vi "PPMS_CREA_SECUENCIA_OLD.vi"(8 "error in (no error)":errorcluster) -> (0 "error out":errorcluster, 1 "Total":string[](array[string]), 2 "Pasos":i32, 3 "Secuencia":string[](array[string]))   [LabVIEW 2017]
uses:
  <vilib>/Utility/file.llb/Read From Spreadsheet File (string).vi
panel:
  out "subArray2D":string[][](array[string])
  out "Seq scans":string[](array[string])
  out "Seq final":string[](array[string])
  out "Seq inicial":string[](array[string])
  out "idxScanTi":i16
  out "idxScanFi":i16
  out "idxScanFf":i16
  out "idxScanTf":i16
  out "Array2D":string[][](array[string])
  out "Scan T":bool
  out "Scan F":bool
  in  "Salir":bool
  in  "Borra linea":bool
  in  "Grabar":bool
  in  "Cargar":bool
  out "SequenceFile":path
  in  "Command line (double click)":i32(listbox) caption="Válvulas"
  in  "Secuencia":i32(listbox)=-1
  # "Septiembre 2019 V1.2  a-sslcdms"
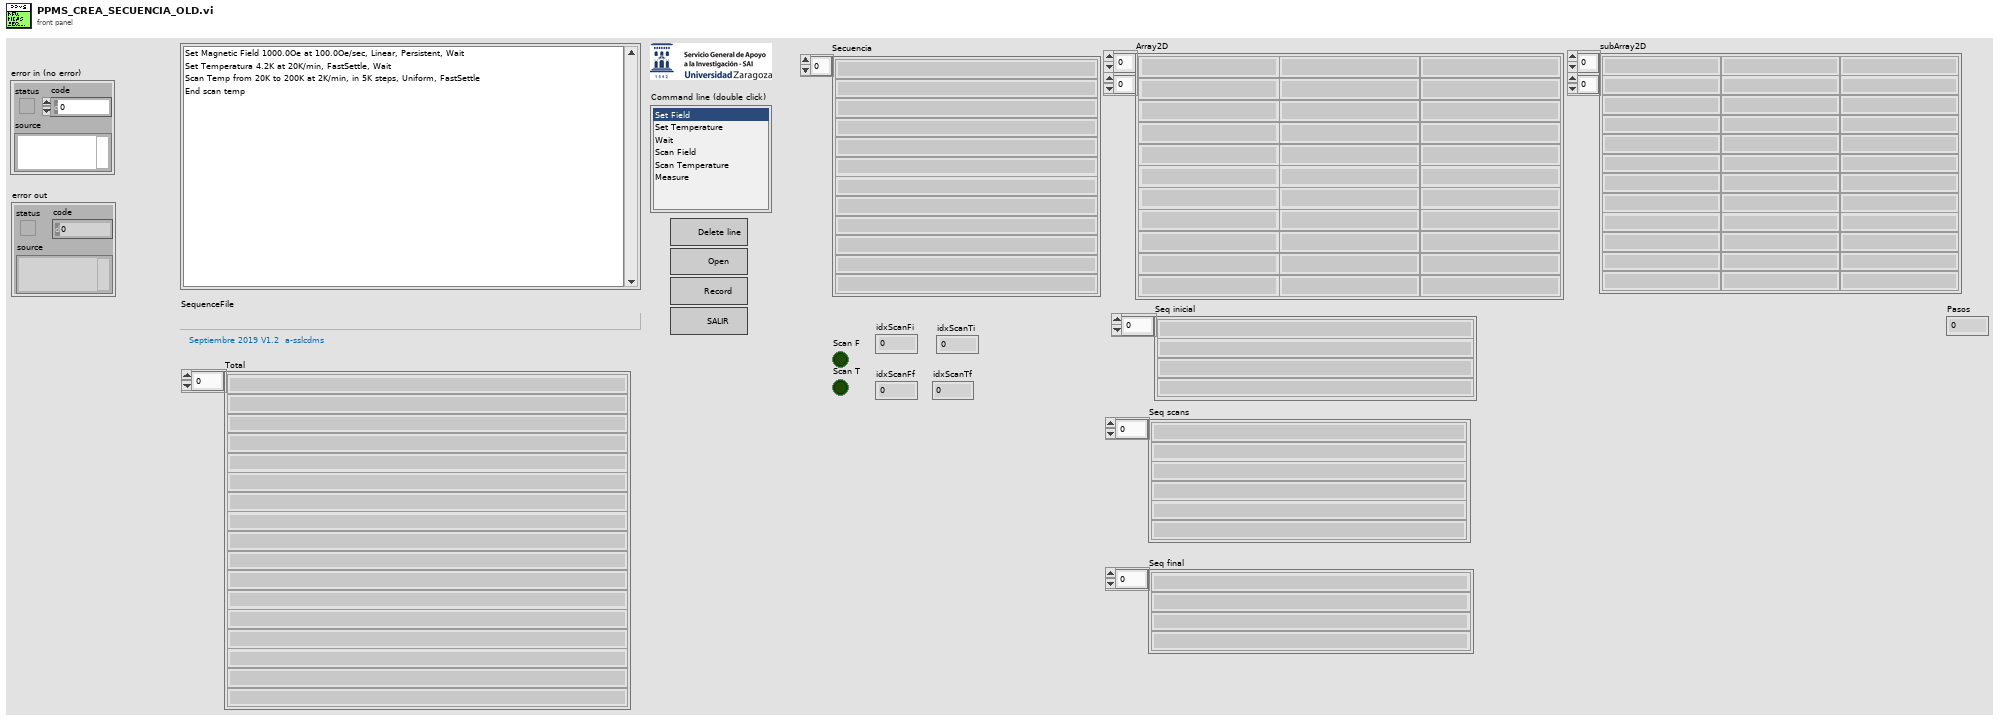
[diagram p1: front panel]
types:
  T1 = enum16{"open", "open or create", "create or replace", "create", "open (read only)"}
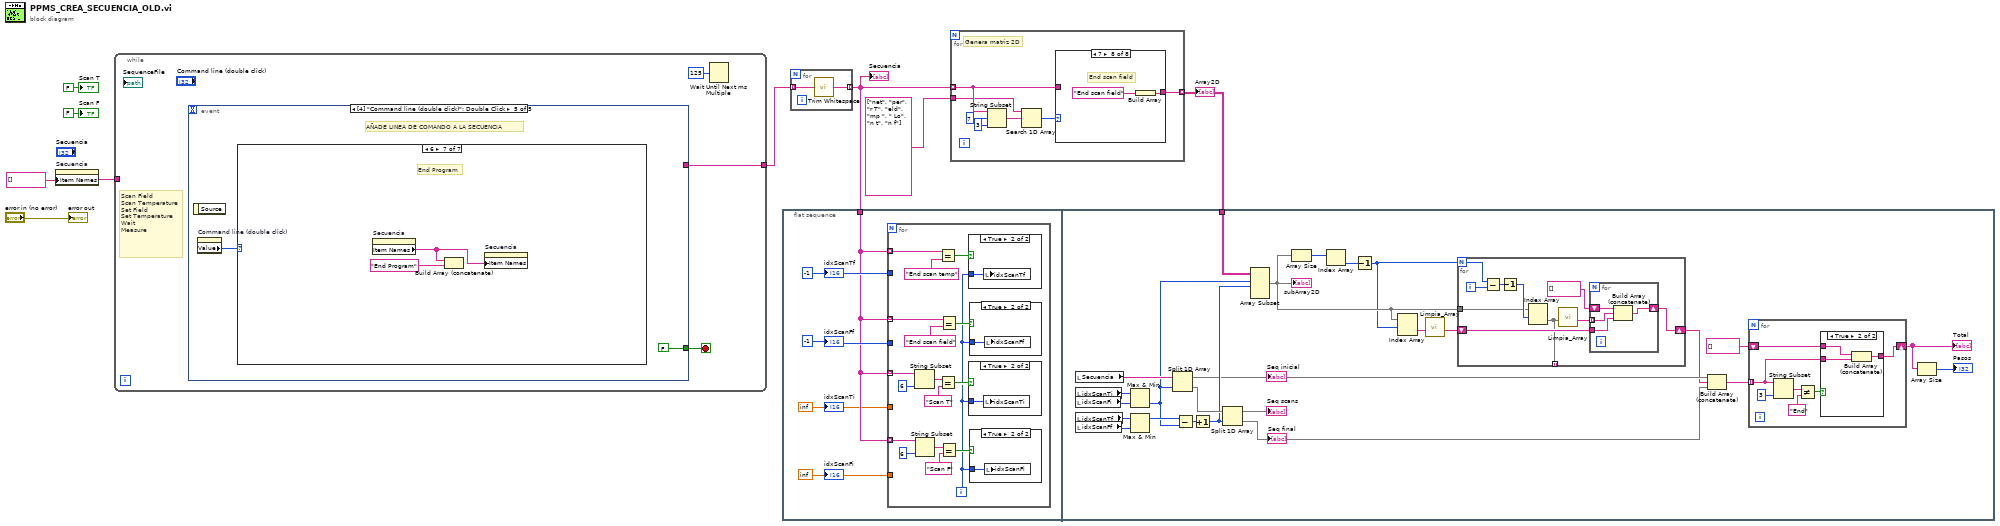
[diagram p0: block diagram]
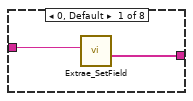
[diagram p7: hidden frame]
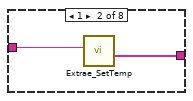
[diagram p8: hidden frame]
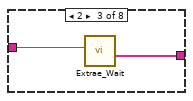
[diagram p9: hidden frame]
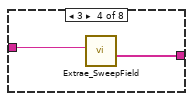
[diagram p10: hidden frame]
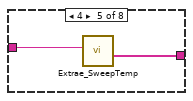
[diagram p11: hidden frame]
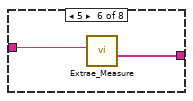
[diagram p12: hidden frame]
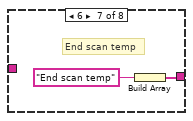
[diagram p13: hidden frame]
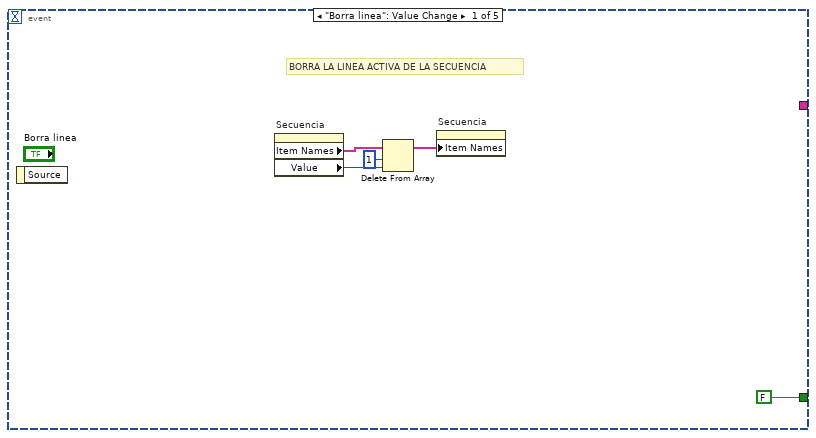
[diagram p14: hidden frame]
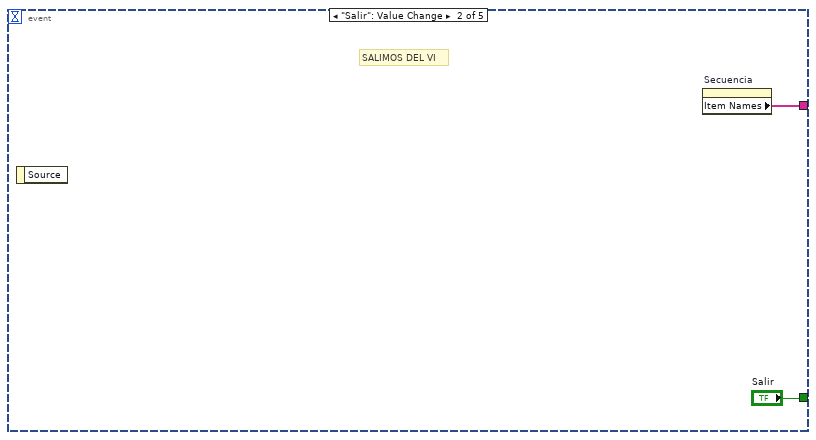
[diagram p15: hidden frame]
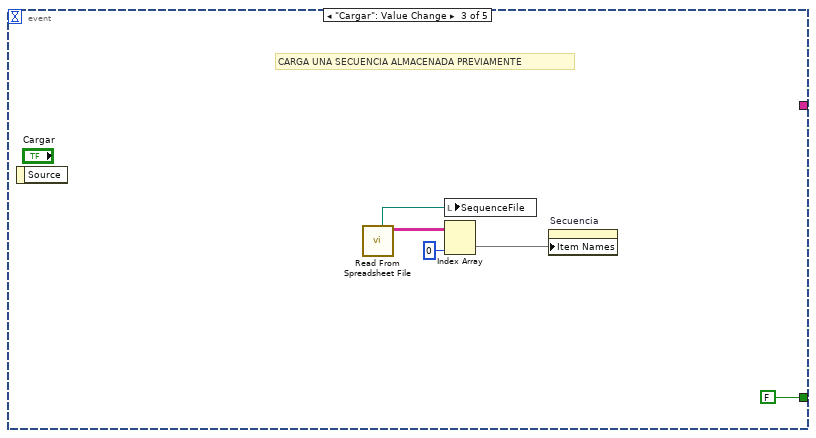
[diagram p16: hidden frame]
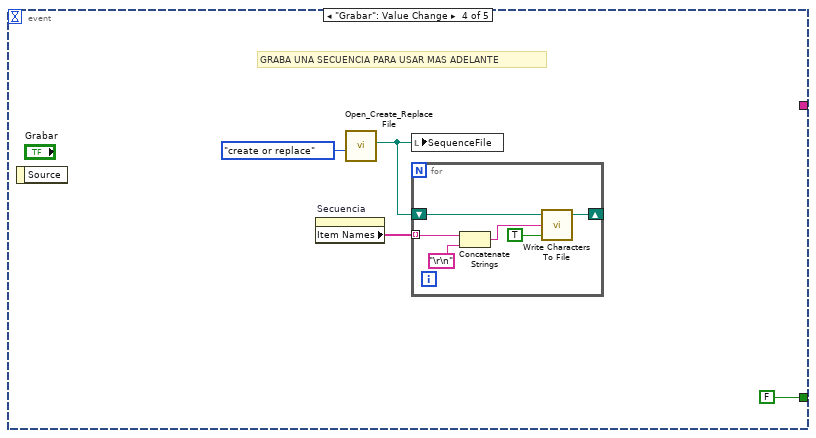
[diagram p17: hidden frame]
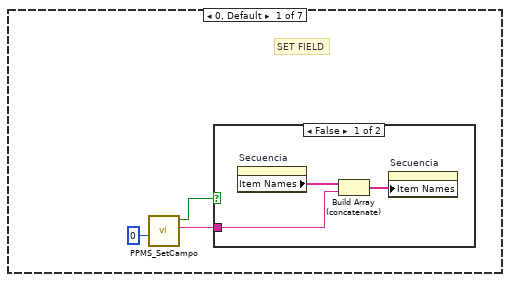
[diagram p18: hidden frame]
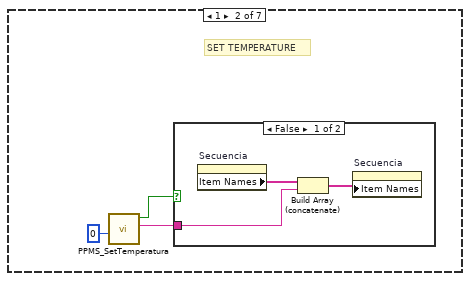
[diagram p20: hidden frame]
diagram:
  w8 = string[] [] ("Item Names")
  n1 = property on="Secuencia" class="LstBox (strict)"("Item Names"=w8) -> ()  [unwired: 2 in, 2 out]
  n2 = while {
    tunnel: w8 -> [_]
    tunnel: [w9] -> w3
    stop <- w10 stop-if-true
    # "Scan Field\nScan Temperature\nSet Field\nSet Temperature\nWait\nMeasure"
    n3 = event shown="[4] \"Command line (double click)\": Double Click" {
      selector: _ -> [_ _ _ _ _]
      dyn-events: _ -> [_ _ _ _ _]
      timeout: _ -> [_ _ _ _ _]
      tunnel: [FALSE ("Salir") "Salir" FALSE ("Salir") FALSE ("Salir") FALSE ("Salir")] -> w10
      tunnel: [_ w17 _ _ _] -> w9
      event "Borra linea": Value Change {
        # "BORRA LA LINEA ACTIVA DE LA SECUENCIA"
        n4 = event-data() -> ()  [unwired: 1 in, 1 out]
        n5 = property on="Secuencia" class="LstBox (strict)"() -> ("Item Names"=w16:string[], "Value"=w15:i32)  [unwired: 2 in, 2 out]
        n6 = Delete From Array(array=w16, length=1, index=w15) -> (array with subset deleted=w13:string[])  [unwired: 1 out]
        n7 = property on="Secuencia" class="LstBox (strict)"("Item Names"=w13) -> ()  [unwired: 2 in, 2 out]
      }
      event "Salir": Value Change {
        # "SALIMOS DEL VI"
        n8 = event-data() -> ()  [unwired: 1 in, 1 out]
        n9 = property on="Secuencia" class="LstBox (strict)"() -> ("Item Names"=w17:string[])  [unwired: 2 in, 2 out]
      }
      event "Cargar": Value Change {
        # "CARGA UNA SECUENCIA ALMACENADA PREVIAMENTE"
        n10 = event-data() -> ()  [unwired: 1 in, 1 out]
        n11 = call-poly <vilib>:"Read From Spreadsheet File.vi"() -> ("all rows"=w21:string[][], "new file path (Not A Path if cancelled)"=w22:path)  [unwired: 7 in, 3 out]
        n12 = local write "SequenceFile"(w22) -> ()
        n13 = Index Array(array=w21, index (col)=0 ("disabled index (col)")) -> (element=w19:string[])  [unwired: 1 in]
        n14 = property on="Secuencia" class="LstBox (strict)"("Item Names"=w19) -> ()  [unwired: 2 in, 2 out]
      }
      event "Grabar": Value Change {
        # "GRABA UNA SECUENCIA PARA USAR MAS ADELANTE"
        n15 = event-data() -> ()  [unwired: 1 in, 1 out]
        n16 = property on="Secuencia" class="LstBox (strict)"() -> ("Item Names"=w27:string[])  [unwired: 2 in, 2 out]
        n17 = call <vilib>:"Open_Create_Replace File.vi"("function (open:0)"=T1."create or replace") -> ("new file path"=w24:path)  [unwired: 7 in, 3 out]
        n18 = local write "SequenceFile"(w24) -> ()
        n19 = for {
          tunnel: w27 -> [w30] mode=indexing
          shift-right: [w32] -> _
          shift-left: w24 -> [w33]
          n20 = Concatenate Strings(w30, "\r\n") -> (w29:string)
          n21 = call <vilib>:"Write Characters To File.vi"("append to file? (new file:F)"=TRUE, "character string"=w29, "file path (dialog if empty)"=w33) -> ("new file path (Not A Path if cancelled)"=w32:path)  [unwired: 2 in]
        }
      }
      event "Command line (double click)": Double Click {
        # "AÑADE LINEA DE COMANDO A LA SECUENCIA"
        n22 = event-data() -> ()  [unwired: 1 in, 1 out]
        n23 = property on="Command line (double click)" class="LstBox (strict)"() -> ("Value"=w34:i32)  [unwired: 2 in, 2 out]
        n24 = case shown="6" w34 {
          frame 0, Default {
            # "SET FIELD"
            n25 = call "PPMS_SetCampo.vi"("Index"=i8 0) -> ("resulting string 1"=w37:string, "Cancelled?"=w38:bool)  [unwired: 6 in, 1 out]
            n26 = case shown="False" w38 {
              tunnel: w37 -> [w39 _]
              frame False {
                n27 = property on="Secuencia" class="LstBox (strict)"() -> ("Item Names"=w40:string[])  [unwired: 2 in, 2 out]
                n28 = Build Array (concatenate)(w40, w39) -> (w41:string[])
                n29 = property on="Secuencia" class="LstBox (strict)"("Item Names"=w41) -> ()  [unwired: 2 in, 2 out]
              }
              frame True {
              }
            }
          }
          frame 1 {
            # "SET TEMPERATURE"
            n30 = call "PPMS_SetTemperatura.vi"("Index"=i8 0) -> ("resulting string 1"=w43:string, "Cancelled?"=w44:bool)  [unwired: 6 in, 1 out]
            n31 = case shown="False" w44 {
              tunnel: w43 -> [w45 _]
              frame False {
                n32 = property on="Secuencia" class="LstBox (strict)"() -> ("Item Names"=w47:string[])  [unwired: 2 in, 2 out]
                n33 = Build Array (concatenate)(w47, w45) -> (w46:string[])
                n34 = property on="Secuencia" class="LstBox (strict)"("Item Names"=w46) -> ()  [unwired: 2 in, 2 out]
              }
              frame True {
              }
            }
          }
          frame 2 {
            # "WAIT CASE"
            n35 = call "PPMS_Wait.vi"("Index"=i8 0) -> ("resulting string 1"=w49:string, "Cancelled?"=w50:bool)  [unwired: 6 in, 1 out]
            n36 = case shown="False" w50 {
              tunnel: w49 -> [w54 _]
              frame False {
                n37 = property on="Secuencia" class="LstBox (strict)"() -> ("Item Names"=w53:string[])  [unwired: 2 in, 2 out]
                n38 = Build Array(w54) -> (w51:string[])
                n39 = Build Array (concatenate)(w53, w51) -> (w52:string[])
                n40 = property on="Secuencia" class="LstBox (strict)"("Item Names"=w52) -> ()  [unwired: 2 in, 2 out]
              }
              frame True {
              }
            }
          }
          frame 3 {
            # "SCAN FIELD"
            n41 = local read "Scan F"() -> (w55:bool)
            n42 = case shown="False" w55 {
              frame False {
                n43 = local read "Scan T"() -> (w58:bool)
                n44 = Select(t=i8 2 ("Index"), s=w58, f=i8 0 ("Index")) -> (s? t:f=w57:i8)
                n45 = local write "Scan F"(TRUE ("Scan T")) -> ()
                n46 = call "PPMS_ScanCampo.vi"("Index"=w57) -> ("resulting string 2"=w62:string, "resulting string 1"=w63:string, "Cancelled?"=w61:bool)  [unwired: 5 in, 1 out]
                n47 = case shown="False" w61 {
                  tunnel: w63 -> [w68 _]
                  tunnel: w62 -> [w67 _]
                  frame False {
                    n48 = property on="Secuencia" class="LstBox (strict)"() -> ("Item Names"=w66:string[])  [unwired: 2 in, 2 out]
                    n49 = Build Array(w68, w67) -> (w65:string[])
                    n50 = Build Array (concatenate)(w66, w65) -> (w64:string[])
                    n51 = property on="Secuencia" class="LstBox (strict)"("Item Names"=w64) -> ()  [unwired: 2 in, 2 out]
                  }
                  frame True {
                  }
                }
              }
              frame True {
                n52 = One Button Dialog(message="Solo esta permitido\nun scan de campo por secuencia") -> ()  [unwired: 1 in, 1 out]
              }
            }
          }
          frame 4 {
            # "SCAN TEMPERATURE"
            n53 = local read "Scan T"() -> (w70:bool)
            n54 = case shown="False" w70 {
              frame False {
                n55 = local read "Scan F"() -> (w72:bool)
                n56 = local write "Scan T"(TRUE ("Scan T")) -> ()
                n57 = Select(t=i8 2 ("Index"), s=w72, f=i8 0 ("Index")) -> (s? t:f=w71:i8)
                n58 = call "PPMS_ScanTemperatura.vi"("Index"=w71) -> ("resulting string 2"=w76:string, "resulting string 1"=w77:string, "Cancelled?"=w78:bool)  [unwired: 5 in, 1 out]
                n59 = case shown="False" w78 {
                  tunnel: w77 -> [w83 _]
                  tunnel: w76 -> [w82 _]
                  frame False {
                    n60 = property on="Secuencia" class="LstBox (strict)"() -> ("Item Names"=w81:string[])  [unwired: 2 in, 2 out]
                    n61 = Build Array(w83, w82) -> (w80:string[])
                    n62 = Build Array (concatenate)(w81, w80) -> (w79:string[])
                    n63 = property on="Secuencia" class="LstBox (strict)"("Item Names"=w79) -> ()  [unwired: 2 in, 2 out]
                  }
                  frame True {
                  }
                }
              }
              frame True {
                n64 = One Button Dialog(message="Solo esta permitido\nun scan de temperatura por secuencia") -> ()  [unwired: 1 in, 1 out]
              }
            }
          }
          frame 5 {
            # "MEASURE CASE"
            n65 = local read "Scan T"() -> (w90:bool)
            n66 = local read "Scan F"() -> (w91:bool)
            n67 = Select(t=i8 2 ("Index"), s=w90, f=i8 0 ("Index")) -> (s? t:f=w86:i8)
            n68 = Select(t=i8 2 ("Index"), s=w91, f=i8 0 ("Index")) -> (s? t:f=w87:i8)
            n69 = Add(x=w87, y=w86) -> (x+y=w85:i8)
            n70 = call "PPMS_Measure.vi"("Index"=w85) -> ("resulting string 1"=w94:string, "Cancelled?"=w95:bool)  [unwired: 6 in, 1 out]
            n71 = case shown="False" w95 {
              tunnel: w94 -> [w99 _]
              frame False {
                n72 = property on="Secuencia" class="LstBox (strict)"() -> ("Item Names"=w97:string[])  [unwired: 2 in, 2 out]
                n73 = Build Array(w99) -> (w96:string[])
                n74 = Build Array (concatenate)(w97, w96) -> (w98:string[])
                n75 = property on="Secuencia" class="LstBox (strict)"("Item Names"=w98) -> ()  [unwired: 2 in, 2 out]
              }
              frame True {
              }
            }
          }
          frame 6 {
            # "End Program"
            n76 = property on="Secuencia" class="LstBox (strict)"() -> ("Item Names"=w100:string[])  [unwired: 2 in, 2 out]
            n77 = Build Array (concatenate)(w100, "End Program" ("message")) -> ()  [unwired: 1 out]
            n78 = property on="Secuencia" class="LstBox (strict)"("Item Names"=w100) -> ()  [unwired: 2 in, 2 out]
          }
        }
      }
    }
    n79 = Wait Until Next ms Multiple(millisecond multiple=u32 125) -> ()  [unwired: 1 out]
  }
  n80 = flat-sequence {
    tunnel: w2 -> [w104]
    tunnel: w1 -> [w143]
    frame #0 {
      w102 = inf
      w103 = inf
      w105 = i16 -1 ("idxScanT")
      w106 = i16 -1 ("idxScanT")
      n81 = for {
        tunnel: w104 -> [w113] mode=indexing
        tunnel: w106 -> [_]
        tunnel: w104 -> [w112] mode=indexing
        tunnel: w105 -> [_]
        tunnel: w104 -> [w110] mode=indexing
        tunnel: w104 -> [w109] mode=indexing
        tunnel: w102 -> [_]
        tunnel: w103 -> [_]
        i -> [w115]
        n82 = String Subset(string=w110, length (rest)=6 ("length (rest)")) -> (substring=w107:string)  [unwired: 1 in]
        n83 = String Subset(string=w109, length (rest)=6 ("length (rest)")) -> (substring=w108:string)  [unwired: 1 in]
        n84 = Equal?(x=w113, y="End scan temp" ("trimmed string")) -> (x = y?=w122:bool)
        n85 = Equal?(x=w107, y="Scan T" ("trimmed string")) -> (x = y?=w117:bool)
        n86 = Equal?(x=w112, y="End scan field" ("trimmed string")) -> (x = y?=w121:bool)
        n87 = Equal?(x=w108, y="Scan F" ("trimmed string")) -> (x = y?=w118:bool)
        n88 = case shown="True" w122 {
          tunnel: w115 -> [_ w127]
          frame False {
          }
          frame True {
            n89 = local write "idxScanTf"(w127) -> ()
          }
        }
        n90 = case shown="True" w117 {
          tunnel: w115 -> [_ w125]
          frame False {
          }
          frame True {
            n91 = local write "idxScanTi"(w125) -> ()
          }
        }
        n92 = case shown="True" w121 {
          tunnel: w115 -> [_ w126]
          frame False {
          }
          frame True {
            n93 = local write "idxScanFf"(w126) -> ()
          }
        }
        n94 = case shown="True" w118 {
          tunnel: w115 -> [_ w124]
          frame False {
          }
          frame True {
            n95 = local write "idxScanFi"(w124) -> ()
          }
        }
      }
      "idxScanTf" <- w106
      "idxScanFf" <- w105
      "idxScanTi" <- w103
      "idxScanFi" <- w102
    }
    frame #1 {
      n96 = local read "Secuencia"() -> (w152:string[])
      n97 = local read "idxScanTi"() -> (w151:i16)
      n98 = local read "idxScanFi"() -> (w150:i16)
      n99 = local read "idxScanTf"() -> (w148:i16)
      n100 = local read "idxScanFf"() -> (w149:i16)
      n101 = Max & Min(x=w151, y=w150) -> (min(x,y)=w142:i16)  [unwired: 1 out]
      n102 = Max & Min(x=w148, y=w149) -> (max(x,y)=w145:i16)  [unwired: 1 out]
      n103 = Split 1D Array(array=w152, index=w142) -> (first subarray=w133:string[], second subarray=w146:string[])
      "Seq inicial" <- w133
      n104 = Subtract(x=w145, y=w142) -> (x-y=w144:i16)
      n105 = Increment(x=w144) -> (x+1=w141:i16)
      n106 = Split 1D Array(array=w146, index=w141) -> (first subarray=→"Seq scans":string[], second subarray=w134:string[])
      "Seq final" <- w134
      n107 = Array Subset(array=w143, index (row)=w142, length (row)=w141) -> (w138:string[][])  [unwired: 2 in]
      "subArray2D" <- w138
      n108 = Array Size(array=w138) -> (size(s)=w137:i32[])
      n109 = Index Array(array=w137) -> (element=w136:i32)  [unwired: 1 in]
      n110 = Decrement(x=w136) -> (x-1=w135:i32)
      n111 = Index Array(array=w138, index (row)=w135) -> (element=w139:string[])  [unwired: 1 in]
      n112 = call "Limpia_Array.vi"("Array in"=w139) -> ("Array out"=w140:string[])  [unwired: 10 in]
      n113 = for {
        N: w135 -> [w173]
        tunnel: w138 -> [w170]
        shift-right: [w166] -> w132
        shift-left: w140 -> [w167]
        tunnel: [w164] -> _ mode=indexing
        i -> [w172]
        n114 = Subtract(x=w173, y=w172) -> (x-y=w169:i32)
        n115 = Decrement(x=w169) -> (x-1=w171:i32)
        n116 = Index Array(array=w170, index (row)=w171) -> (element=w164:string[])  [unwired: 1 in]
        n117 = call "Limpia_Array.vi"("Array in"=w164) -> ("Array out"=w165:string[])  [unwired: 10 in]
        n118 = for {
          tunnel: w165 -> [w176] mode=indexing
          shift-right: [w174] -> w166
          shift-left: string[] [] -> [w177]
          tunnel: w167 -> [w175]
          n119 = Build Array (concatenate)(w177, w176, w175) -> (w174:string[])
        }
      }
      n120 = Build Array (concatenate)(w133, w132, w134) -> (w131:string[])
      n121 = for {
        tunnel: w131 -> [w153] mode=indexing
        shift-right: [w155] -> w129
        shift-left: string[] [] -> [w156]
        n122 = String Subset(string=w153, length (rest)=3 ("length (rest)")) -> (substring=w159:string)  [unwired: 1 in]
        n123 = Not Equal?(x=w159, y="End" ("trimmed string")) -> (x != y?=w154:bool)
        n124 = case shown="True" w154 {
          tunnel: w156 -> [w160 w163]
          tunnel: [w160 w162] -> w155
          tunnel: w153 -> [_ w161]
          frame False {
          }
          frame True {
            n125 = Build Array (concatenate)(w163, w161) -> (w162:string[])
          }
        }
      }
      "Total" <- w129
      n126 = Array Size(array=w129) -> (size(s)=→"Pasos":i32)
    }
  }
  n127 = for {
    tunnel: w3 -> [w179] mode=indexing
    tunnel: [w178] -> w2 mode=indexing
    n128 = call <vilib>:"Trim Whitespace.vi"("string"=w179) -> ("trimmed string"=w178:string)  [unwired: 1 in]
  }
  "Secuencia" <- w2
  n129 = for {
    tunnel: w2 -> [w181] mode=indexing
    tunnel: [w182] -> w1 mode=indexing
    tunnel: string[] ["net", "per", "r T", "eld", "mp ", " Lo", "n t", "n f"] ("Array") -> [w180]
    # "Genera matriz 2D"
    n130 = String Subset(string=w181, offset (0)=7, length (rest)=3 ("length (rest)")) -> (substring=w184:string)
    n131 = Search 1D Array(1D array=w180, element=w184) -> (index of element=w183:i32)  [unwired: 1 in]
    n132 = case shown="7" w183 {
      tunnel: w181 -> [w188 w190 w192 w194 w196 w198 _ _]
      tunnel: [w187 w189 w191 w193 w195 w197 w199 w201] -> w182
      frame 0, Default {
        n133 = call "Extrae_SetField.vi"("String"=w188) -> ("Array"=w187:string[])  [unwired: 10 in]
      }
      frame 1 {
        n134 = call "Extrae_SetTemp.vi"("String"=w190) -> ("Array"=w189:string[])  [unwired: 10 in]
      }
      frame 2 {
        n135 = call "Extrae_Wait.vi"("String"=w192) -> ("Array"=w191:string[])  [unwired: 10 in]
      }
      frame 3 {
        n136 = call "Extrae_SweepField.vi"("F string"=w194) -> ("Array F"=w193:string[])  [unwired: 10 in]
      }
      frame 4 {
        n137 = call "Extrae_SweepTemp.vi"("T string"=w196) -> ("Array T"=w195:string[])  [unwired: 10 in]
      }
      frame 5 {
        n138 = call "Extrae_Measure.vi"("String"=w198) -> ("Array"=w197:string[])  [unwired: 10 in]
      }
      frame 6 {
        # "End scan temp"
        n139 = Build Array("End scan temp" ("trimmed string")) -> (w199:string[])
      }
      frame 7 {
        # "End scan field"
        n140 = Build Array("End scan field" ("trimmed string")) -> (w201:string[])
      }
    }
  }
  "Array2D" <- w1
  "error out" <- "error in (no error)"
  "Scan F" <- FALSE ("Loop H")
  "Scan T" <- FALSE ("Loop T")
